vi "Long word to bytes.vi"(5 "Litt/BigEnd":bool, 7 "Index":i32, 8 "U32":u32, 9 "Image Data in":u8[](array[numeric])) -> (1 "Index+4":i32, 3 "Image Data out":u8[](array[numeric]))   [LabVIEW 2015, in "Tiff reader.lvlib"]
doc: "Converts word into 4 bytes."
uses:
  Tiff reader.lvlib
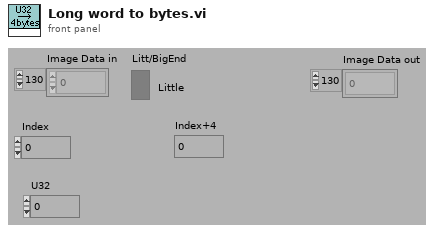
[diagram p1: front panel]
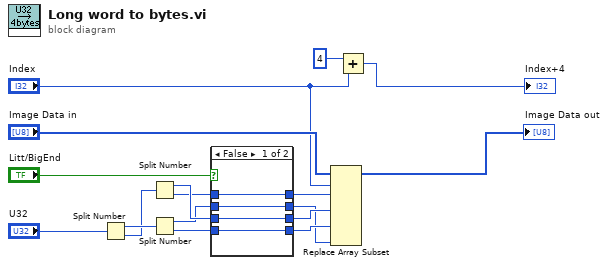
[diagram p0: block diagram]
diagram:
  n1 = Split Number(x="U32") -> (hi(x)=w10:u16, lo(x)=w9:u16)
  n2 = Split Number(x=w9) -> (hi(x)=w8:u8, lo(x)=w7:u8)
  n3 = Split Number(x=w10) -> (hi(x)=w6:u8, lo(x)=w5:u8)
  n4 = case shown="False" "Litt/BigEnd" {
    tunnel: [w21 w22] -> w14
    tunnel: w7 -> [w21 w25]
    tunnel: [w20 w23] -> w13
    tunnel: w8 -> [w20 w24]
    tunnel: [w19 w24] -> w12
    tunnel: w5 -> [w19 w23]
    tunnel: [w18 w25] -> w11
    tunnel: w6 -> [w18 w22]
    frame False {
    }
    frame True {
    }
  }
  n5 = Replace Array Subset "Replace Array Subset"(array="Image Data in", new element #1=w14, index #1="Index", new element #2=w13, new element #3=w12, new element #4=w11) -> (→"Image Data out":u8[])  [unwired: 3 in]
  n6 = Add(x=4, y="Index") -> (x+y=→"Index+4":i32)
